vi "test Drive.vi"() -> ()   [LabVIEW 2018]
uses:
  <vilib>/Rock Robotics/WPI/ThirdParty/REV Robotics/SPARK MAX/Typedef/Spark MAX Control Type.ctl
panel:
  in  "PID Constants":T1={"P Gain"=0.0, "I Gain"=0.0, "D Gain"=0.0, "F Gain"=0.0, "I Zone"=0.0, "Min Output"=-1.0, "Max Output"=1.0} {"Max Output" min=-1.0 max=1.0 step=0.01; "Min Output" min=-1.0 max=1.0 step=0.01; "I Zone" step=0.01; "F Gain" step=0.01; "D Gain" step=0.01; "I Gain" step=0.01; "P Gain" min=0.0 step=0.01}
  out "PID Chart":T2(graph)
  in  "Setpoint":dbl(slide) scale=-5700.0..5700.0
  in  "Drive Speed":dbl
  # "Click here to set max"
  # "Click here to set min"
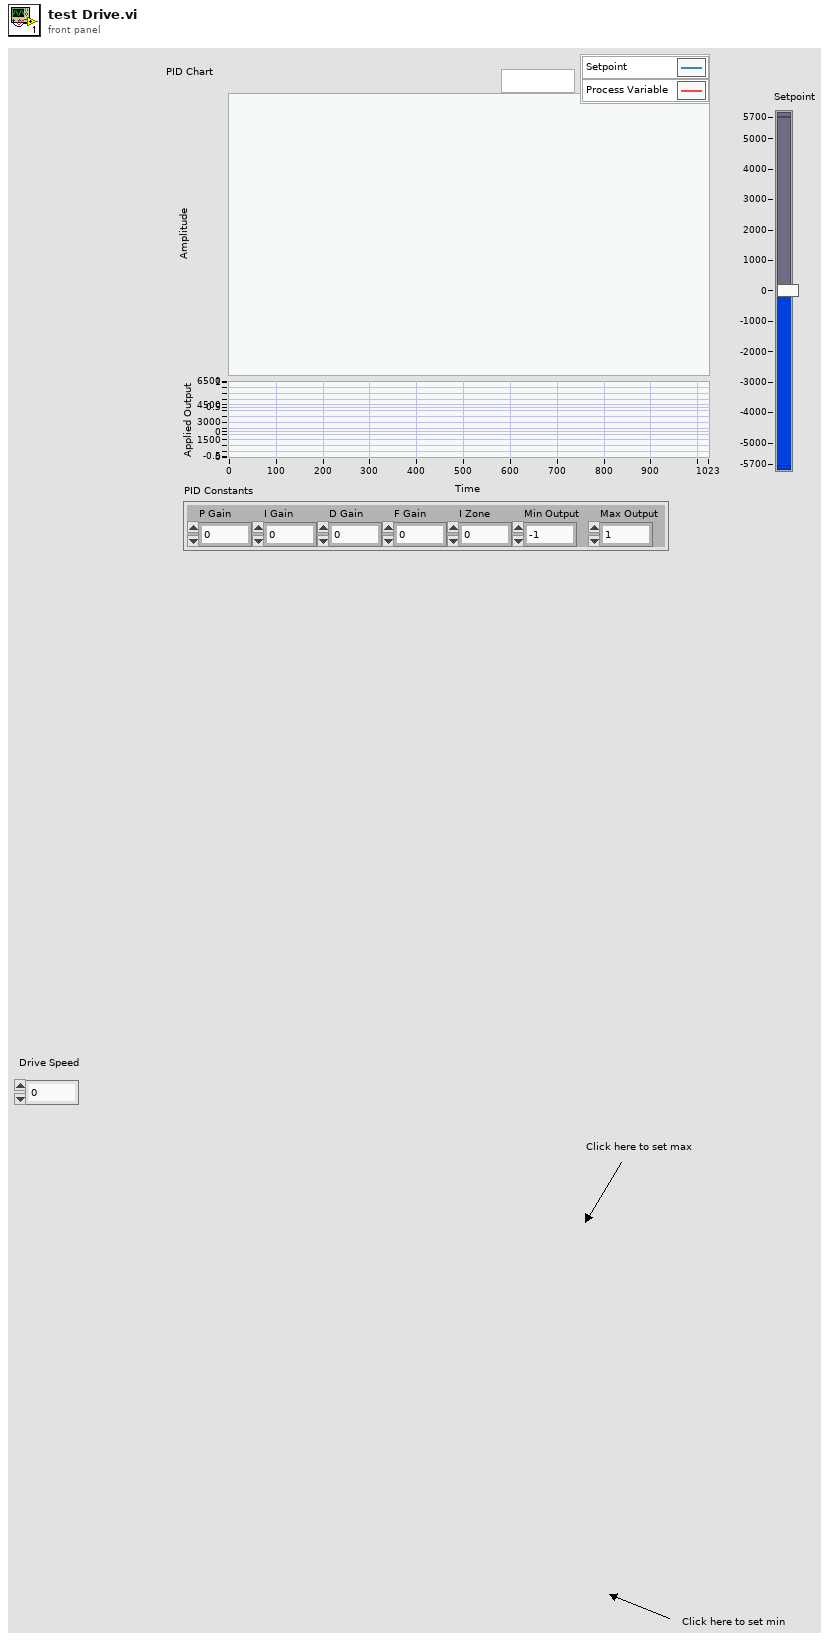
[diagram p1: front panel]
types:
  T1 = cluster{"P Gain":dbl, "I Gain":dbl, "D Gain":dbl, "F Gain":dbl, "I Zone":dbl, "Min Output":dbl, "Max Output":dbl}
  T2 = cluster{"Sensor Velocity":dbl, "Setpoint":dbl, "Applied Output":dbl}
  T3 = typedef "Spark MAX Control Type.ctl" = enum16{"Percent VBus", "Voltage", "Velocity", "Position", "Smart Motion", "Current", "Smart Velocity"}
  T4 = typedef "WPI_MotorControlDeviceRef.ctl" = cluster{"DeviceStatus":errorcluster, "Type":T5, "PWM":cluster{"PWM Channel":T6, "DeadBand":T7}, "CAN":cluster{"Device Number":u8, "SetOutput VI Ref":variant, "GetOutput VI Ref":variant, "Enable VI Ref":variant, "Disable VI Ref":variant, "Data":variant}, "Invert":bool, "DIO PWM":cluster{"PWM \"Enable\" Channel":T6, "DIOChannel":T8, "PWM Rate":dbl}}
  T5 = typedef "WPI_MotorControlType.ctl" = enum16{"PWM", "CAN", "DIO PWM"}
  T6 = typedef "FPGA_DIOPWMChannel.ctl" = enum8{"PWM 0", "PWM 1", "PWM 2", "PWM 3", "PWM 4", "PWM 5", "PWM 6", "PWM 7", "PWM 8", "PWM 9", "PWM MXP 0", "PWM MXP 1", "PWM MXP 2", "PWM MXP 3", "PWM MXP 4", "PWM MXP 5", "PWM MXP 6", "PWM MXP 7", "PWM MXP 8", "PWM MXP 9", "Invalid"}
  T7 = typedef "WPI_PWMDeadband.ctl" = cluster{"Name":string, "maxPositivePwm":i32, "minPositivePwm":i32, "centerPwm":i32, "maxNegativePwm":i32, "minNegativePwm":i32, "angularRange":u16}
  T8 = typedef "FPGA_DIOChannel.ctl" = enum8{"DIO 0", "DIO 1", "DIO 2", "DIO 3", "DIO 4", "DIO 5", "DIO 6", "DIO 7", "DIO 8", "DIO 9", "DIO MXP 0", "DIO MXP 1", "DIO MXP 2", "DIO MXP 3", "DIO MXP 4", "DIO MXP 5", "DIO MXP 6", "DIO MXP 7", "DIO MXP 8", "DIO MXP 9", "DIO MXP 10", "DIO MXP 11", "DIO MXP 12", "DIO MXP 13", "DIO MXP 14", "DIO MXP 15", "SPI Port CS1", "SPI Port CS2", "SPI Port CS3", "SPI Port MISO", "SPI Port MOSI", "Invalid"}
  T9 = cluster{"P Gain":bool, "I Gain":bool, "D Gain":bool, "F Gain":bool, "I Zone":bool, "Min Output":bool, "Max Output":bool}
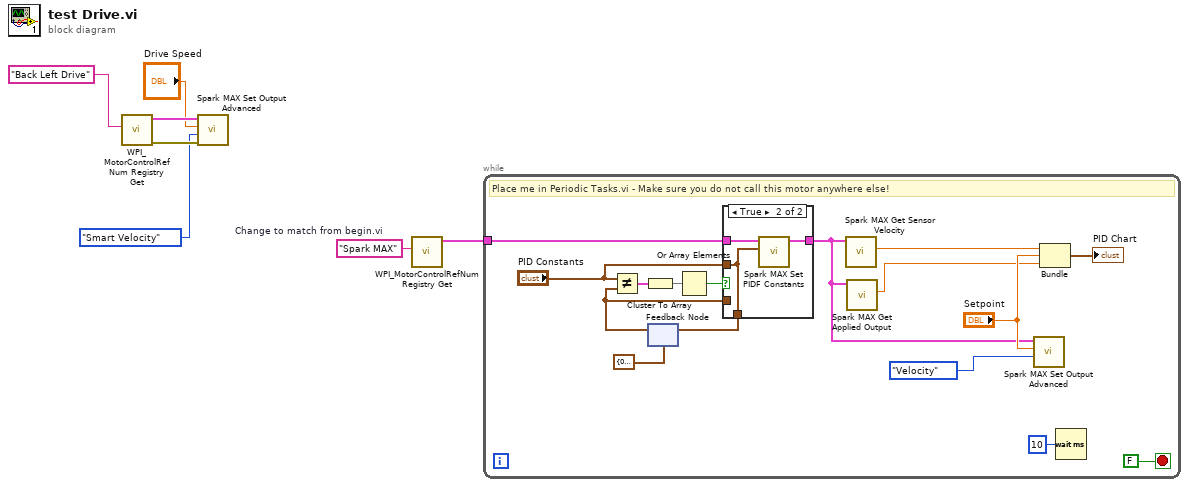
[diagram p0: block diagram]
diagram:
  w1 = "Spark MAX"  # Change to match from begin.vi
  n1 = call <vilib>:"WPI_MotorControlRefNum Registry Get.vi"("refnum name"="Back Left Drive") -> ("error out"=w7:errorcluster, "MotorControlDevRef"=w6:T4)  [unwired: 9 in]
  n2 = call <vilib>:"Spark MAX Set Output Advanced.vi"("error in (no error)"=w7, "Control Mode"=Spark_MAX_Control_Type."Smart Velocity", "Setpoint"="Drive Speed", "MotorControlDevRef"=w6) -> ()  [unwired: 6 in, 2 out]
  n3 = call <vilib>:"WPI_MotorControlRefNum Registry Get.vi"("refnum name"=w1) -> ("MotorControlDevRef"=w2:T4)  [unwired: 9 in, 1 out]
  n4 = while {
    tunnel: w2 -> [w13]
    stop <- FALSE stop-if-true
    # "Place me in Periodic Tasks.vi - Make sure you do not call this motor anywhere else!"
    n5 = feedback #1(T1 {"P Gain"=0.0, "I Gain"=0.0, "D Gain"=0.0, "F Gain"=0.0, "I Zone"=0.0, "Min Output"=0.0, "Max Output"=0.0} ("PID Constants")) -> (w20:T1)
    n6 = Not Equal?(x="PID Constants", y=w20) -> (x != y?=w14:T9)
    n7 = Cluster To Array(cluster=w14) -> (array=w15:bool[])
    n8 = Or Array Elements(Boolean array=w15) -> (logical OR=w17:bool)
    n9 = case shown="True" w17 {
      tunnel: w13 -> [w24 w28]
      tunnel: "PID Constants" -> [_ w26]
      tunnel: [w25 w26] -> w19
      tunnel: w20 -> [w25 _]
      tunnel: [w24 w27] -> w8
      frame False {
      }
      frame True {
        n10 = call <vilib>:"Spark MAX Set PIDF Constants.vi"("PID Constants"=w26, "MotorControlDeviceRef"=w28) -> ("MotorControlDeviceRef"=w27:T4)  [unwired: 8 in, 1 out]
      }
    }
    n11 = feedback-in #1(w19) -> ()
    n12 = call <vilib>:"Spark MAX Get Sensor Velocity.vi"("MotorControlDevRef in"=w8) -> ("Sensor Velocity"=w10:dbl)  [unwired: 7 in, 3 out]
    n13 = call <vilib>:"Spark MAX Get Applied Output.vi"("MotorControlDevRef in"=w8) -> ("Applied Output"=w9:dbl)  [unwired: 7 in, 3 out]
    n14 = call <vilib>:"Spark MAX Set Output Advanced.vi"("Control Mode"=Spark_MAX_Control_Type."Velocity", "Setpoint"="Setpoint", "MotorControlDevRef"=w8) -> ()  [unwired: 7 in, 2 out]
    n15 = Bundle("Sensor Velocity"=w10, "Setpoint"="Setpoint", "Applied Output"=w9) -> (→"PID Chart":T2)  [unwired: 1 in]
    n16 = Wait (ms)(milliseconds to wait=u32 10) -> ()  [unwired: 1 out]
  }
